vi "Set Boolean Colourbox Colour.vi"(8 "error in (no error)":errorcluster, 10 "Boolean State":T1, 11 "ColorBox in":refnum<vi>) -> (0 "error out":errorcluster)   [LabVIEW 2015, in "Utility.lvlib"]
uses:
  Utility.lvlib
  Typedef/Boolean Indicator State.ctl
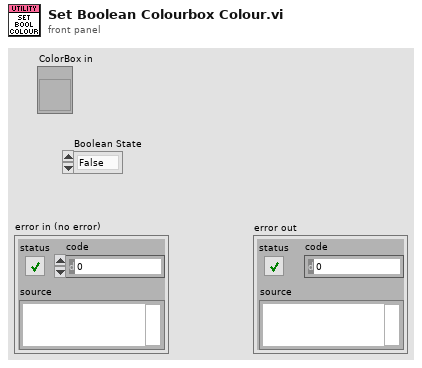
[diagram p1: front panel]
types:
  T1 = typedef "Utility.lvlib/Boolean Indicator State.ctl" = enum16{"False", "True", "Error"}
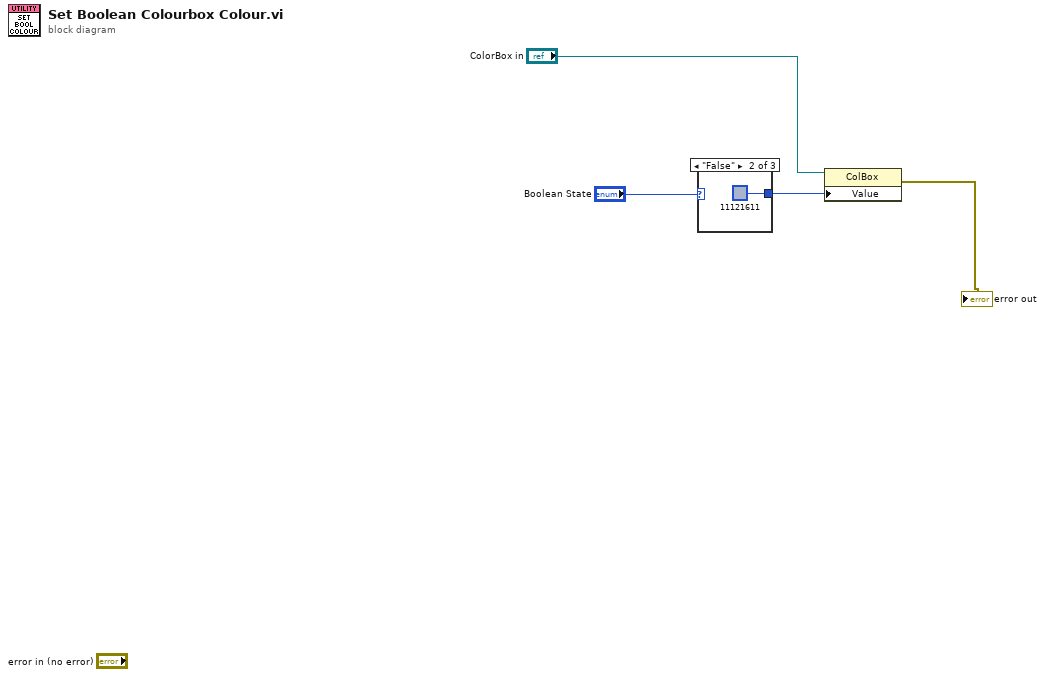
[diagram p0: block diagram]
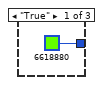
[diagram p2: hidden frame]
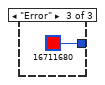
[diagram p3: hidden frame]
diagram:
  n1 = case shown="\"False\"" "Boolean State" {
    tunnel: [u32 6618880 u32 11121611 u32 16711680] -> w2
    frame "True" {
    }
    frame "False" {
    }
    frame "Error" {
    }
  }
  n2 = property class="ColBox"(reference="ColorBox in", "Value"=w2) -> (error out=→"error out":errorcluster)  [unwired: 1 in, 1 out]
